vi "Server Thread Handle Message (Heartbeat).vi"(3 "error in":errorcluster, 4 "Heartbeat Message":T2={"type"="heartbeat", "message"="{}"}, 5 "Timestamp":dbl format="%#_13g", 6 "Server Thread":T1) -> (0 "error out":errorcluster, 1 "Heartbeat Message":T2={"type"="heartbeat", "message"="{}"}, 2 "Server Thread":T1)   [LabVIEW 2016]
uses:
  Messages/Heartbeat/Heartbeat Message.ctl
  Server Thread.ctl
  Messages/Heartbeat/Heartbeat Message to JSON.vi
  <vilib>/Rock Robotics/Network Tables/NT Write Number.vi
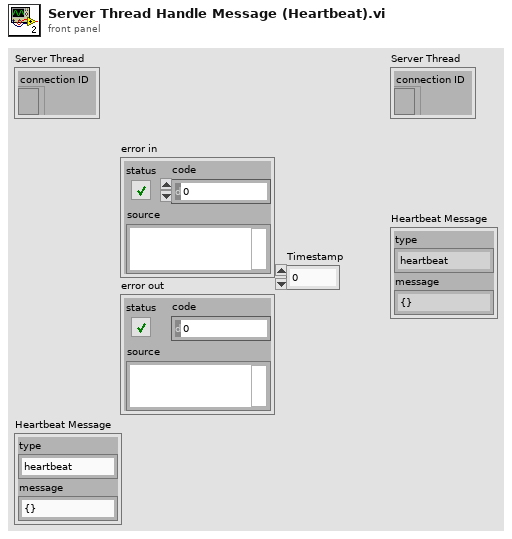
[diagram p1: front panel]
types:
  T1 = typedef "Server Thread.ctl" = cluster{"connection ID":refnum<k5>}
  T2 = typedef "Heartbeat Message.ctl" = cluster{"type":string, "message":string}
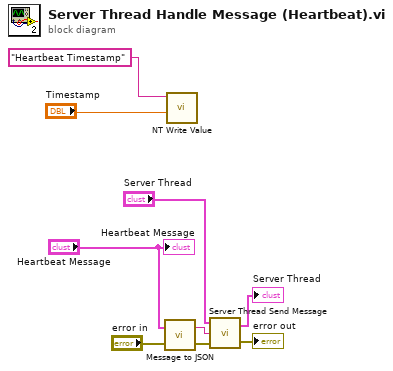
[diagram p0: block diagram]
diagram:
  n1 = call-poly "Message to JSON.vi"("error in"="error in", "Heartbeat Message"="Heartbeat Message") -> ("error out"=w7:errorcluster, "JSON string"=w8:string)
  n2 = call-poly <vilib>:"NT Write Value.vi"("Numeric"="Timestamp", "Name"="Heartbeat Timestamp") -> ()  [unwired: 9 in, 1 out]
  n3 = call "Server Thread Send Message.vi"("error in"=w7, "JSON string"=w8, "Server Thread"="Server Thread") -> ("error out"=→"error out":errorcluster, "Server Thread"=→"Server Thread":T1)
  "Heartbeat Message" <- "Heartbeat Message"
